vi "Write Characters with check.vi"(2 "String to Write":string, 3 "Call EnFlo Error Handler?":bool=TRUE, 4 "file (use dialog)":path) -> (0 "error out":errorcluster)   [LabVIEW 2022 SP3]
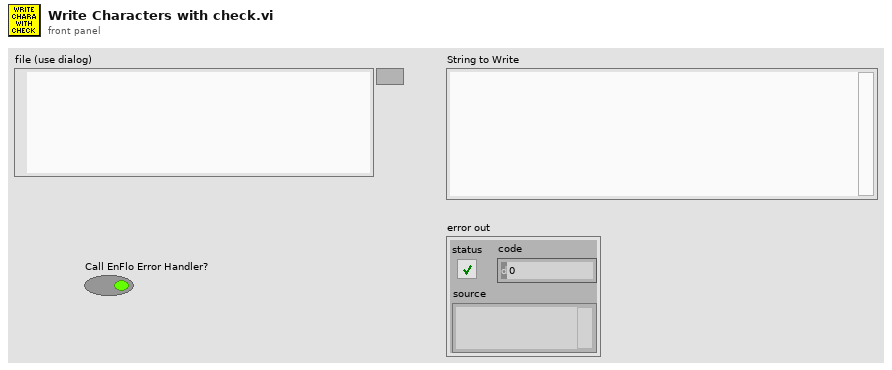
[diagram p1: front panel]
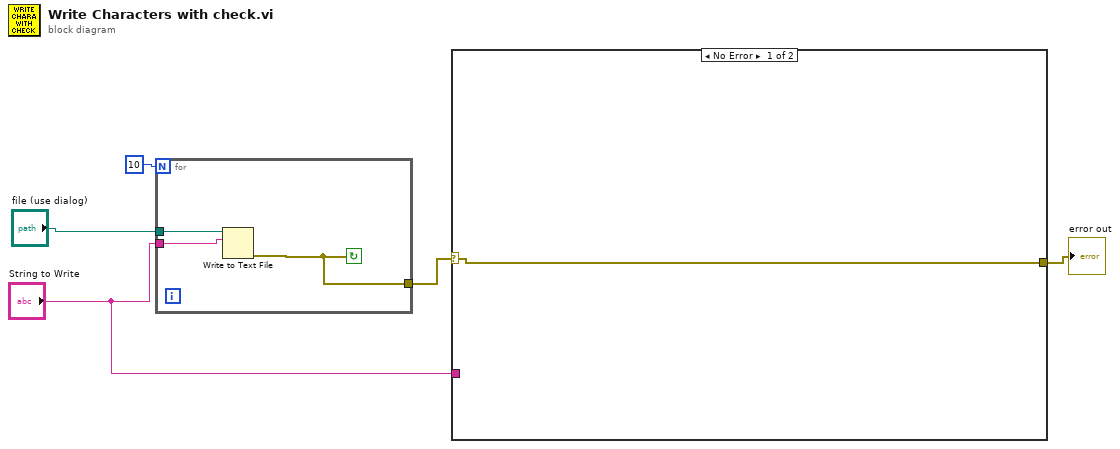
[diagram p0: block diagram]
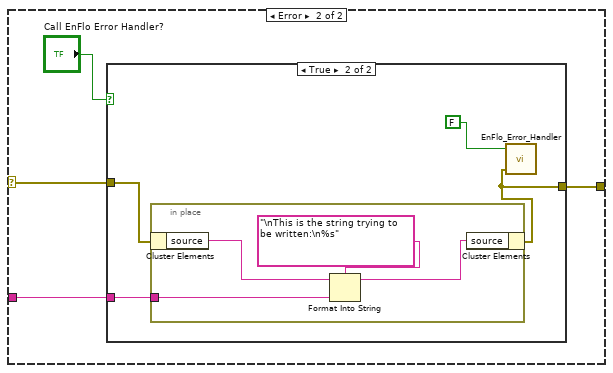
[diagram p2: hidden frame]
diagram:
  n1 = for {
    N: 10 -> [_]
    tunnel: "file (use dialog)" -> [w8]
    tunnel: [w6] -> w3
    tunnel: "String to Write" -> [w7]
    stop <- w6 continue-if-true
    n2 = Write to Text File(file (use dialog)=w8, text=w7) -> (error out=w6:errorcluster)  [unwired: 2 in, 2 out]
  }
  n3 = case shown="No Error" w3 {
    selector: w3 -> [w9 w13]
    tunnel: "String to Write" -> [_ w11]
    tunnel: [w9 w10] -> w1
    frame No Error {
    }
    frame Error {
      n4 = case shown="True" "Call EnFlo Error Handler?" {
        tunnel: w13 -> [w14 w17]
        tunnel: w11 -> [_ w16]
        tunnel: [w14 w15] -> w10
        frame False {
        }
        frame True {
          n5 = in-place {
            in-place-border: w16 -> [w21]
            n6 = in-place-cluster #1(w17) -> ("source"=w22:string)
            n7 = Format Into String(format string="\nThis is the string trying to be written:\n%s", initial string=w22, w21) -> (resulting string=w20:string)  [unwired: 1 in, 1 out]
            n8 = in-place-cluster #1("source"=w20) -> (w15:errorcluster)
          }
          n9 = call "EnFlo_Error_Handler.vi"("error in (no error)"=w15, "Dialog Box (F)"=FALSE) -> ()  [unwired: 2 in, 2 out]
        }
      }
    }
  }
  "error out" <- w1
